vi "xijk_set_help_position.vi"(11 "tab in":u32) -> (3 "position left out":i32)   [LabVIEW 2009]
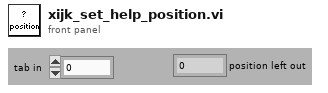
[diagram p1: front panel]
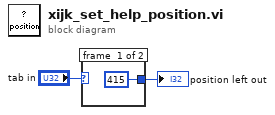
[diagram p0: block diagram]
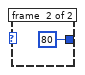
[diagram p2: hidden frame]
diagram:
  n1 = case shown="5..12" "tab in" {
    tunnel: [415 ("position left out") 80 ("position left out")] -> w1
    frame #0 {
    }
    frame #1 {
    }
  }
  "position left out" <- w1
